vi "FrameNames to StateNames.vi"(11 "FrameNames":string[](array[string])) -> (3 "Array of Strings":string[](array[string]))   [LabVIEW 2017, in "CSM-Helper.lvclass"]
uses:
  CSM-Helper.lvclass
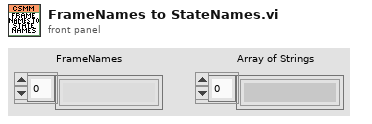
[diagram p1: front panel]
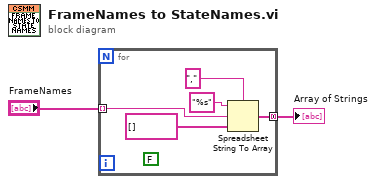
[diagram p0: block diagram]
diagram:
  n1 = for {
    tunnel: "FrameNames" -> [w7] mode=indexing
    tunnel: [w5] -> w2 mode=concatenating
    (unwired) FALSE ("ignore duplicate delimiters? (F=No)")
    n2 = Spreadsheet String To Array(delimiter (Tab)=",", format string="%s", spreadsheet string=w7, array type (2D Dbl)=string[] [] ("Array of Strings")) -> (array=w5:string[])
  }
  "Array of Strings" <- w2
